vi "Parse Key Press.vi"(8 "PlatMods":T1, 9 "Mods":cluster{"Num Pad":bool, "Menu Key":bool}, 10 "ScanCode":i16, 11 "VKey":T2) -> (3 "Key Pressed":string)   [LabVIEW 2018, in "User Interface.lvlib"]
doc: "Converts key press info into a string representing the keys pressed. Output is in the form [MODIFIER + ][NUM_]SCANCODE.\n\nFor example:\nA\nSHIFT + A\nSHIFT + CTRL + A\nNUM_ENTER"
uses:
  User Interface.lvlib
  <vilib>/event_ctls.llb/eventvkey.ctl
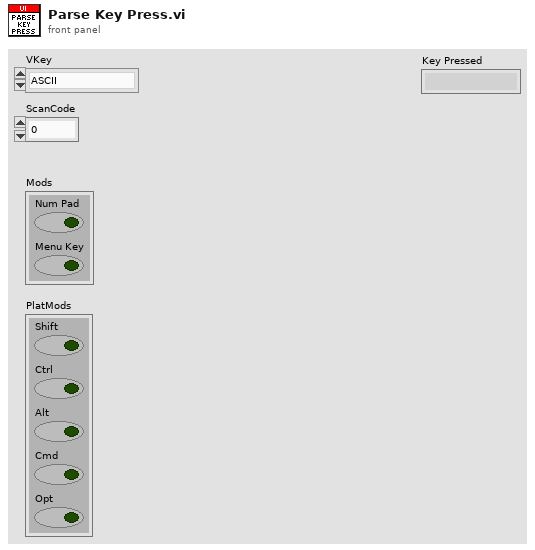
[diagram p1: front panel]
types:
  T1 = cluster{"Shift":bool, "Ctrl":bool, "Alt":bool, "Cmd":bool, "Opt":bool}
  T2 = typedef "eventvkey.ctl" = enum16{"ASCII", "Enter", "Return", "Shift", "Ctrl", "Alt", "Cmd", "Opt", "Caps", "NumLock", "Clear", "Break", "Up", "Down", "Left", "Right", "Insert", "Delete", "Home", "End", "PageUp", "PageDown", "Escape", "Help", "Pause", "ScrollLock", "F1", "F2", "F3", "F4", "F5", "F6", "F7", "F8", "F9", "F10", "F11", "F12", "F13", "F14", "F15", "F16", "F17", "F18", "F19", "F20", "F21", "F22", "F23", "F24", "Play", "VolumeUp", "VolumeDown", "Mute", "Two Byte Char"}
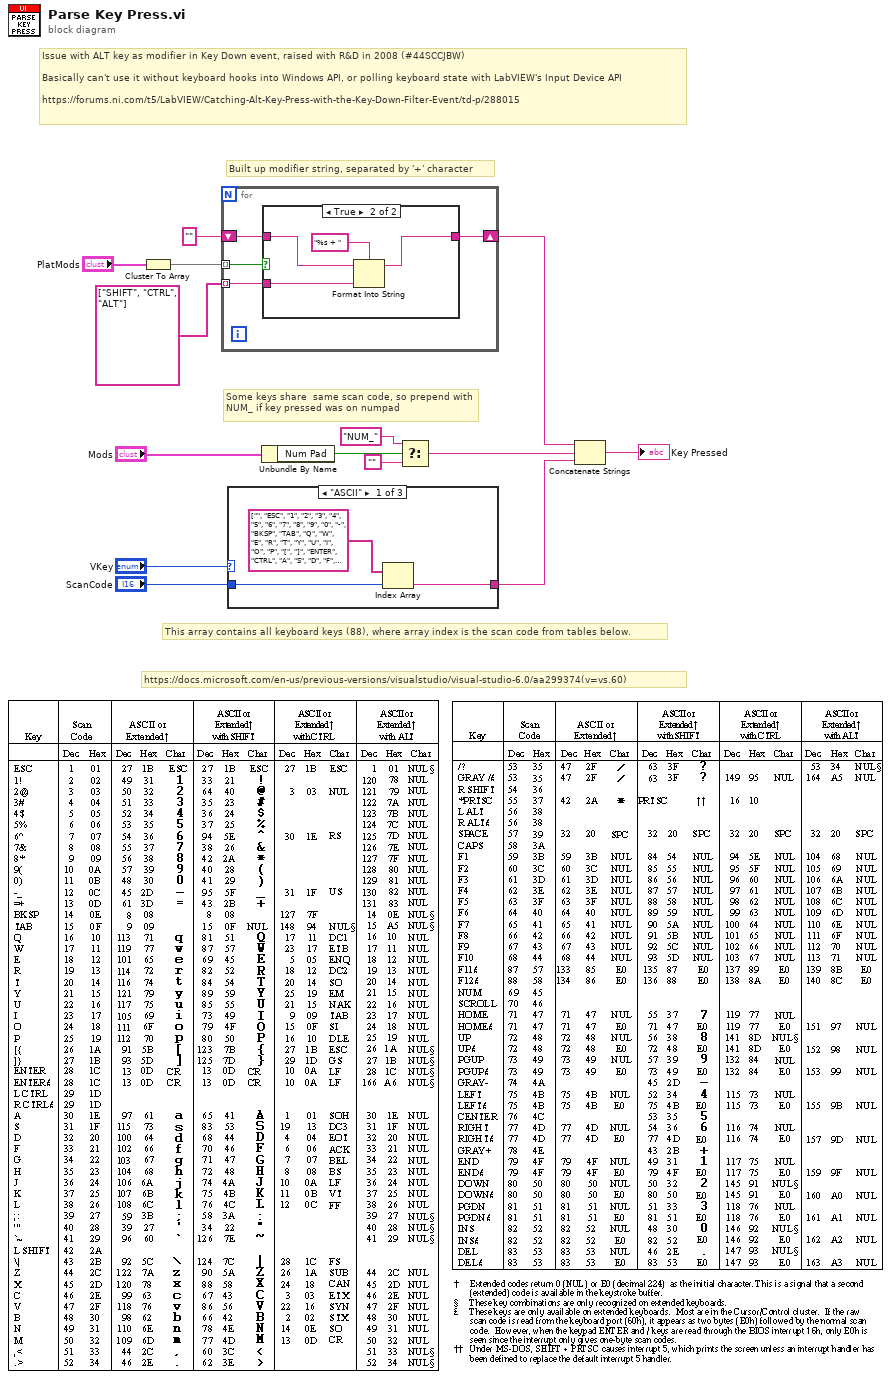
[diagram p0: block diagram]
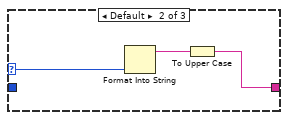
[diagram p2: hidden frame]
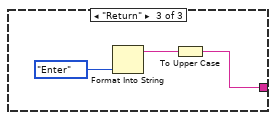
[diagram p3: hidden frame]
diagram:
  # "Issue with ALT key as modifier in Key Down event, raised with R&D in 2008 (#44SCCJBW)\n\nBasically can't use it without keyboard hooks into Windows API, or polling keyboard state with LabVIEW's Input Device API\n\nhttps://forums.ni.com/t5/LabVIEW/Catching-Alt-Key-Press-with-the-Key-Down-Filter-Event/td-p/288015"
  # "https://docs.microsoft.com/en-us/previous-versions/visualstudio/visual-studio-6.0/aa299374(v=vs.60)"
  # "This array contains all keyboard keys (88), where array index is the scan code from tables below."
  # "Some keys share  same scan code, so prepend with NUM_ if key pressed was on numpad"
  # "Built up modifier string, separated by '+' character"
  n1 = Cluster To Array(cluster="PlatMods") -> (array=w14:bool[])
  n2 = for {
    tunnel: w14 -> [w18] mode=indexing
    shift-right: [w15] -> w11
    shift-left: "" -> [w17]
    tunnel: string[] ["SHIFT", "CTRL", "ALT"] -> [w16] mode=indexing
    n3 = case shown="True" w18 {
      tunnel: w17 -> [w19 w21]
      tunnel: w16 -> [_ w23]
      tunnel: [w19 w20] -> w15
      frame False {
      }
      frame True {
        n4 = Format Into String(format string="%s + ", initial string=w21, w23) -> (resulting string=w20:string)  [unwired: 1 in, 1 out]
      }
    }
  }
  n5 = case shown="\"ASCII\"" "VKey" {
    selector: "VKey" -> [_ w29 _]
    tunnel: [w24 w27 w31] -> w7
    tunnel: "ScanCode" -> [w26 _ _]
    frame "ASCII" {
      n6 = Index Array(array=string[] ["", "ESC", "1", "2", "3", "4", "5", "6", "7", "8", "9", "0", "-", "=", "BKSP", "TAB", "Q", "W", "E", "R", "T", "Y", "U", "I", "O", "P", "[", "]", "ENTER", "CTRL", "A", "S", "D", "F", "G", "H", "J", "K", "L", ";", "'", "`", "LSHIFT", "\\", "Z", "X", "C", "V", "B", "N", "M", ",", ".", "/", "RSHIFT", "*", "ALT", "SPACE", "CAPS", "F1", "F2", "F3", "F4", "F5", "F6", "F7", "F8", "F9", "F10", "NUM", "SCROLL", "HOME", "UP", "PGUP", "-", "LEFT", "CENTER", "RIGHT", "+", "END", "DOWN", "PGDN", "INS", "DEL", "", "", "", "F11", "F12"], index=w26) -> (element=w24:string)
    }
    frame Default {
      n7 = Format Into String(w29) -> (resulting string=w28:string)  [unwired: 3 in, 1 out]
      n8 = To Upper Case(1:w28) -> (0:w27:string)
    }
    frame "Return" {
      n9 = Format Into String(eventvkey."Enter" ("input 1")) -> (resulting string=w32:string)  [unwired: 3 in, 1 out]
      n10 = To Upper Case(1:w32) -> (0:w31:string)
    }
  }
  n11 = Unbundle By Name("Mods") -> ("Num Pad"=w8:bool)
  n12 = Select(t="NUM_", s=w8, f="") -> (s? t:f=w6:string)
  n13 = Concatenate Strings(w11, w6, w7) -> (→"Key Pressed":string)
